vi "To File (Ref).vi"(6 "Pretty Print?":bool, 8 "error in (no error)":errorcluster, 10 "JSON Datatype in":refnum<class "JSON Null.lvclass">, 11 "refnum in":refnum<file>) -> (0 "error out":errorcluster, 3 "refnum out":refnum<file>)   [LabVIEW 2016, in "LVJSON.lvlib" / "JSON Helper.lvclass"]
doc: "Saves a JSON instance's data to the given file."
uses:
  JSON Helper.lvclass
  JSON Datatype/JSON Null.lvclass
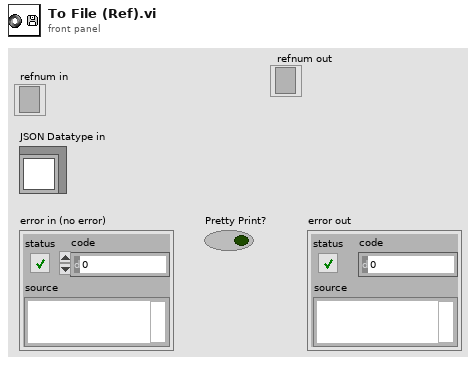
[diagram p1: front panel]
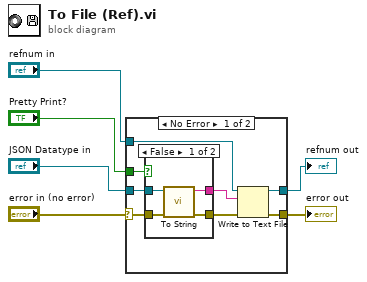
[diagram p0: block diagram]
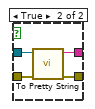
[diagram p2: hidden frame]
diagram:
  n1 = case shown="No Error" "error in (no error)" {
    selector: "error in (no error)" -> [w12 w24]
    tunnel: "JSON Datatype in" -> [w14 _]
    tunnel: [w8 w24] -> w4
    tunnel: "Pretty Print?" -> [w11 _]
    tunnel: "refnum in" -> [w9 w23]
    tunnel: [w7 w23] -> w1
    frame No Error {
      n2 = case shown="False" w11 {
        tunnel: w14 -> [w18 w20]
        tunnel: [w17 w19] -> w13
        tunnel: w12 -> [w16 w21]
        tunnel: [w15 w22] -> w10
        frame False {
          n3 = call-dynamic "To String.vi"("error in (no error)"=w16, "JSON Datatype in"=w18) -> ("error out"=w15:errorcluster, "String"=w17:string)  [unwired: 8 in]
        }
        frame True {
          n4 = call-dynamic "To Pretty String.vi"("error in (no error)"=w21, "JSON Datatype in"=w20) -> ("error out"=w22:errorcluster, "Pretty Print String"=w19:string)  [unwired: 8 in]
        }
      }
      n5 = Write to Text File(file (use dialog)=w9, text=w13, error in=w10) -> (refnum out=w7:refnum<file>, error out=w8:errorcluster)  [unwired: 1 in, 1 out]
    }
    frame Error {
    }
  }
  "error out" <- w4
  "refnum out" <- w1
